vi "sub_NI_Vsion_clamp_copy.vi"(7 "Settings":T3={"Contrast"=40, "Filter width"=4, "Steepness"=2, "Subsampling Ratio"=5, "Show Search Area"=FALSE, "Show Search Lines"=FALSE, "Show Edges Found"=FALSE, "Show Result"=TRUE}, 8 "error in (no error)":errorcluster, 9 "Coordinate System":T5 {"Measurement System"."Axis Reference" items=["Direct", "Indirect"]; "Measurement System"."Angle (deg)" format="%.2f"; "Measurement System"."Origin"."Y" format="%.2f"; "Measurement System"."Origin"."X" format="%.2f"; "Reference System"."Axis Reference" items=["Direct", "Indirect"]; "Reference System"."Angle (deg)" format="%.2f"; "Reference System"."Origin"."Y" format="%.2f"; "Reference System"."Origin"."X" format="%.2f"}, 10 "Rectangle":T6 {"Rotation" format="%.2f"; "Left" scale=0.0..1024.0; "Right" scale=0.0..1024.0}, 11 "Image":T4) -> (0 "error out":errorcluster, 1 "clamp_result":T2 {"ROI Descriptor out"."Contours"."Type" items=["No Selection", "Point", "Line", "Rectangle", "Oval", "Polygon", "Freehand Region", "Annulus", "Unused2", "Unused3", "Broken Line", "Freehand Line", "Rotated Rectangle"]}, 2 "dir-data":cluster{"Distance":sgl, "weight-dir":dbl}, 3 "Image Out":T4, 5 "Edge Coordinates":cluster{"X":sgl, "Y":sgl}[](array[cluster]) {"Y" format="%.2f"; "X" format="%.2f"})   [LabVIEW 2019]
uses:
  <vilib>/vision/Image Controls.llb/IMAQ Image.ctl
  Ctrl/clamp-result_cmd.ctl
  <vilib>/vision/NI_Vision_Development_Module.lvlib
panel:
  out "XY 그래프":cluster{"X":sgl, "Y":sgl}[](graph)
  out "Edge Points":cluster{"X":sgl, "Y":sgl}[](array[cluster])
  out "Elapsed time (ms)":u32
  out "Distance":sgl format="%.2f"
  out "Coordinate System (duplicate)":T5 {"Measurement System"."Axis Reference" items=["Direct", "Indirect"]; "Measurement System"."Angle (deg)" format="%.2f"; "Measurement System"."Origin"."Y" format="%.2f"; "Measurement System"."Origin"."X" format="%.2f"; "Reference System"."Axis Reference" items=["Direct", "Indirect"]; "Reference System"."Angle (deg)" format="%.2f"; "Reference System"."Origin"."Y" format="%.2f"; "Reference System"."Origin"."X" format="%.2f"}
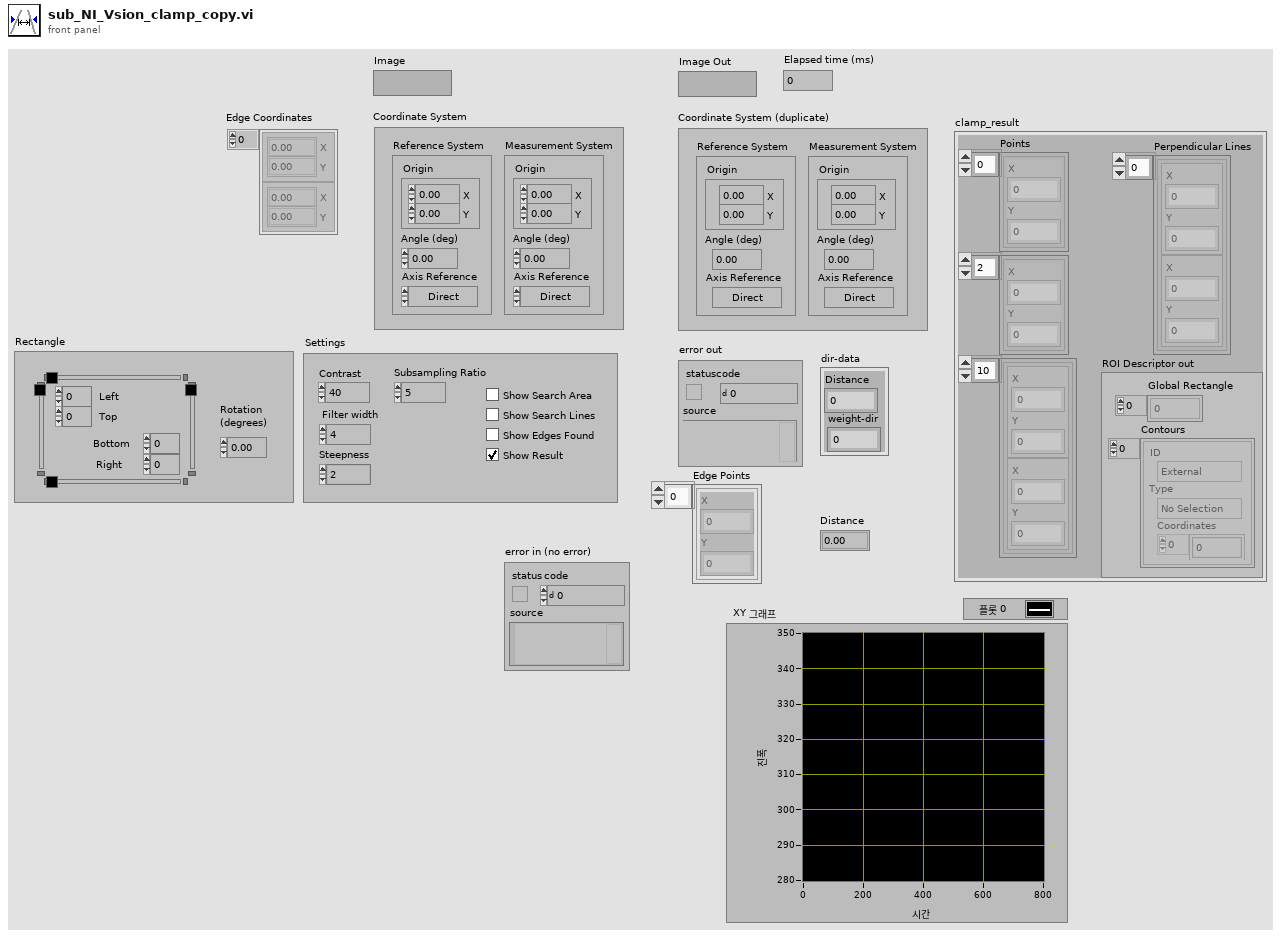
[diagram p1: front panel]
types:
  T1 = typedef "ROI Descriptor" = cluster{"Global Rectangle":i32[], "Contours":cluster{"ID":enum32{"External", "Internal"}, "Type":u32, "Coordinates":i32[]}[]}
  T2 = cluster{"Points":cluster{"X":sgl, "Y":sgl}[], cluster{"X":sgl, "Y":sgl}[], cluster{cluster{"X":sgl, "Y":sgl}, cluster{"X":sgl, "Y":sgl}}[], "Perpendicular Lines":cluster{cluster{"X":sgl, "Y":sgl}, cluster{"X":sgl, "Y":sgl}}[], "ROI Descriptor out":T1}
  T3 = cluster{"Contrast":i32, "Filter width":i32, "Steepness":i32, "Subsampling Ratio":u32, "Show Search Area":bool, "Show Search Lines":bool, "Show Edges Found":bool, "Show Result":bool}
  T4 = typedef "IMAQ Image.ctl" = refnum<image>
  T5 = typedef "IMAQ Coordinate System" = cluster{"Reference System":cluster{"Origin":cluster{"X":sgl, "Y":sgl}, "Angle (deg)":sgl, "Axis Reference":u32}, "Measurement System":cluster{"Origin":cluster{"X":sgl, "Y":sgl}, "Angle (deg)":sgl, "Axis Reference":u32}}
  T6 = typedef "IMAQ Rectangle" = cluster{"Left":i32, "Top":i32, "Right":i32, "Bottom":i32, "Rotation":dbl}
  T7 = typedef "clamp-result_cmd.ctl" = enum16{"write_clamp_overlay-result", "write_center-distance", "write_clamp_result", "write_threshold_result", "read"}
  T8 = cluster{"Origin":cluster{"X":sgl, "Y":sgl}, "Angle (deg)":sgl, "Axis Reference":u32}
  T9 = cluster{"Global Rectangle":i32[], "Contours":cluster{"ID":enum32{"External", "Internal"}, "Type":u32, "Coordinates":i32[]}[]}
  T10 = cluster{"Interpolation Type":enum32{"", "Quadratic", "Cubic Spline"}, "SubPixel Accuracy":enum32{"None", "One Half", "One Third", "One Fourth", "One Fifth", "One Sixth", "One Seventh", "One Eight", "One Ninth", "One Tenth", "One Eleventh", "One Twelveth"}}
  T11 = enum32{"Get First Edge", "Get First + Last Edge", "Get All Edges"}
  T12 = cluster{"Contrast":i32, "Filter width":i32, "Steepness":i32}
  T13 = cluster{cluster{"X":sgl, "Y":sgl}, cluster{"X":sgl, "Y":sgl}}[]
  T14 = cluster{cluster{"X":sgl, "Y":sgl}, cluster{"X":sgl, "Y":sgl}}
  T15 = cluster{"Show Search Area":bool, "Show Search Lines":bool, "Show Edges Found":bool, "Show Result":bool}
  T16 = cluster{"x-center":dbl, "Image Size":cluster{"x":i32, "y":i32}, "Angle deg":sgl, "Threshold Range":cluster{"Lower value":sgl, "Upper value":sgl}}
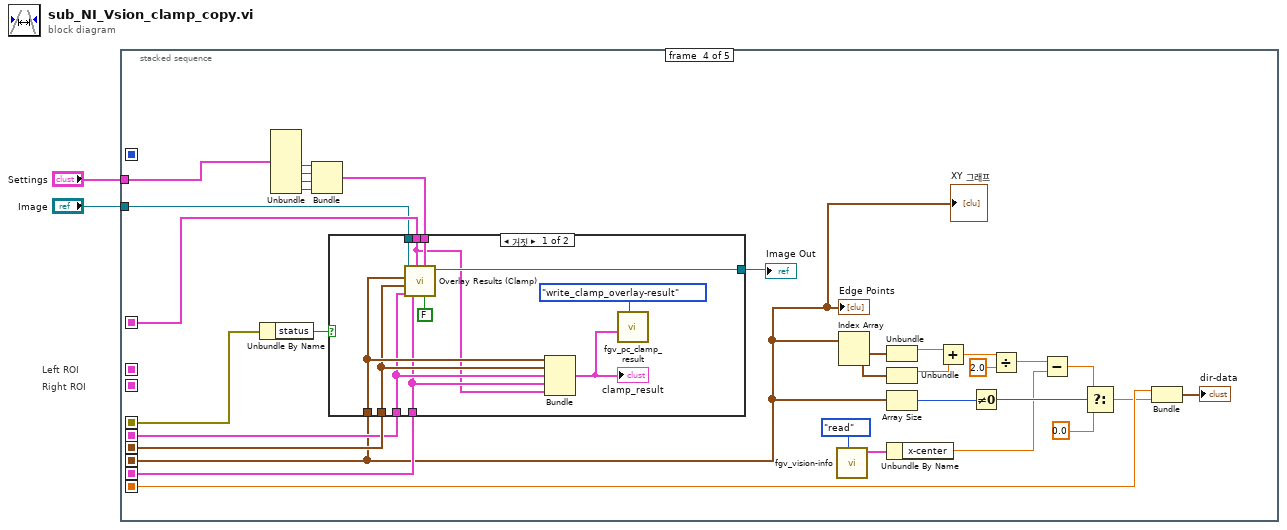
[diagram p0: block diagram]
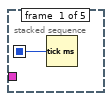
[diagram p2: hidden frame]
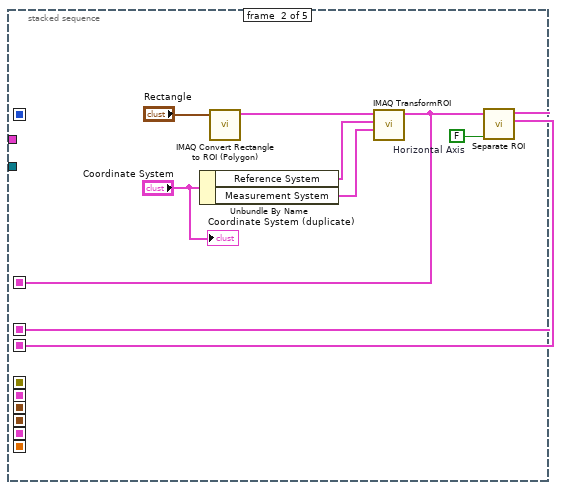
[diagram p3: hidden frame]
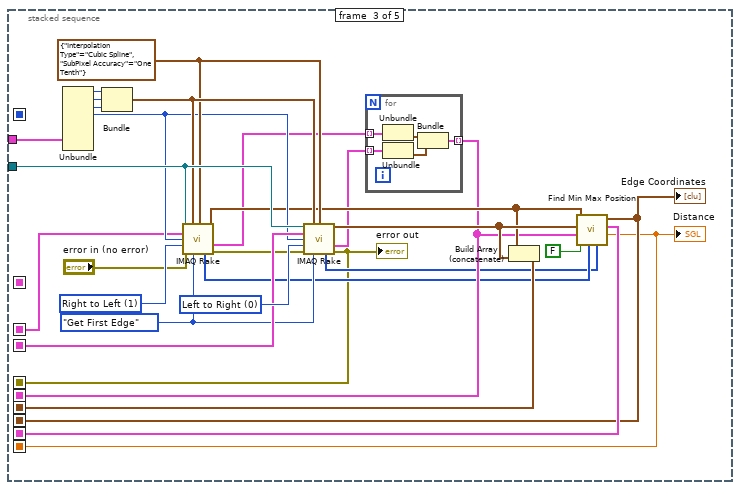
[diagram p4: hidden frame]
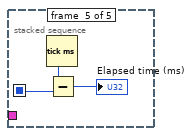
[diagram p6: hidden frame]
diagram:
  # "Right ROI"
  # "Left ROI"
  n1 = stacked-sequence {
    seq-local: [_ _ w33 _ _] -> [_ _ _ w46 _]
    seq-local: [w3 _ _ _ _] -> [_ _ _ _ w92]
    seq-local: [_ _ w34 _ _] -> [_ _ _ w73 _]
    seq-local: [_ _ w20 _ _] -> [_ _ _ w72 _]
    seq-local: [_ _ w37 _ _] -> [_ _ _ w71 _]
    seq-local: [_ w8 _ _ _] -> [_ _ w18 _ _]
    seq-local: [_ w7 _ _ _] -> [_ _ w32 _ _]
    seq-local: [_ w6 _ _ _] -> [_ _ _ w69 _]
    seq-local: [_ _ w14 _ _] -> [_ _ _ w66 _]
    seq-local: [_ _ w13 _ _] -> [_ _ _ w53 _]
    tunnel: "Image" -> [_ _ w30 w68 _]
    tunnel: "Settings" -> [_ _ w17 w50 _]
    frame #0 {
      n2 = Tick Count (ms)() -> (millisecond timer value=w3:u32)
    }
    frame #1 {
      w9 = FALSE  # Horizontal Axis
      # "Find Edges"
      n3 = Unbundle By Name("Coordinate System") -> ("Reference System"=w5:T8, "Measurement System"=w4:T8)
      n4 = call "IMAQ Convert Rectangle to ROI (Polygon)"("Rectangle"="Rectangle") -> ("ROI Descriptor"=w10:T1)  [unwired: 7 in, 2 out]
      n5 = call "IMAQ TransformROI"("New Reference"=w4, "Base Reference"=w5, "ROI Descriptor"=w10) -> ("ROI Descriptor out"=w6:T1)  [unwired: 7 in, 1 out]
      n6 = call <vilib>:"Separate ROI.vi"("Axis"=w9, "ROI Descriptor"=w6) -> ("Right/Bottom ROI"=w7:T9, "Left/Top ROI"=w8:T9)  [unwired: 4 in]
      "Coordinate System (duplicate)" <- "Coordinate System"
    }
    frame #2 {
      w27 = u32 1 items=["Left to Right", "Right to Left", "Top to Bottom", "Bottom to Top"]
      w28 = T10 {"Interpolation Type"=enum."Cubic Spline", "SubPixel Accuracy"=enum."One Tenth"} ("SubPixel Information")
      w22 = T11."Get First Edge" ("Process")
      w35 = u32 0 items=["Left to Right", "Right to Left", "Top to Bottom", "Bottom to Top"]
      # "Find Edges"
      n7 = Unbundle(w17) -> ("Contrast"=w38:i32, "Filter width"=w39:i32, "Steepness"=w40:i32, "Subsampling Ratio"=w25:u32)  [unwired: 4 out]
      n8 = Bundle("Contrast"=w38, "Filter width"=w39, "Steepness"=w40) -> (w29:T12)  [unwired: 1 in]
      n9 = call "IMAQ Rake"("Image"=w30, "Edge Parameters"=w29, "SubPixel Information"=w28, "ROI Descriptor"=w18, "Step Size"=w25, "Scan Direction"=w27, "error in (no error)"="error in (no error)", "Process"=w22) -> ("First Edges"=w23:cluster{"X":sgl, "Y":sgl}[], "Line Coordinates"=w21:T13, "Lines with Edges"=w16:u32[], "error out"=w31:errorcluster)  [unwired: 2 in, 2 out]
      n10 = call "IMAQ Rake"("Image"=w30, "Edge Parameters"=w29, "SubPixel Information"=w28, "ROI Descriptor"=w32, "Step Size"=w25, "Scan Direction"=w35, "error in (no error)"=w31, "Process"=w22) -> ("First Edges"=w24:cluster{"X":sgl, "Y":sgl}[], "Line Coordinates"=w19:T13, "Lines with Edges"=w15:u32[], "error out"=w14:errorcluster)  [unwired: 2 in, 2 out]
      "error out" <- w14
      n11 = for {
        tunnel: w21 -> [w45] mode=indexing
        tunnel: w19 -> [w44] mode=indexing
        tunnel: [w41] -> w20 mode=indexing
        n12 = Unbundle(w45) -> (w43:cluster{"X":sgl, "Y":sgl})  [unwired: 1 out]
        n13 = Unbundle(w44) -> (w42:cluster{"X":sgl, "Y":sgl})  [unwired: 1 out]
        n14 = Bundle(w43, w42) -> (w41:T14)  [unwired: 1 in]
      }
      n15 = Build Array (concatenate)(w23, w24) -> (w34:cluster{"X":sgl, "Y":sgl}[])
      n16 = call <vilib>:"Find Min Max Position.vi"("Lines with Edges (last)"=w15, "Lines with Edges (first)"=w16, "Min / Max"=FALSE, "Search Lines"=w20, "Last Edges"=w24, "First Edges"=w23) -> ("Distance"=w13:sgl, "Perpendicular Lines"=w37:T13, "Points"=w33:cluster{"X":sgl, "Y":sgl}[])  [unwired: 3 in]
      "Edge Coordinates" <- w33
      "Distance" <- w13
    }
    frame #3 {
      # "Update Overlay"
      n17 = Unbundle By Name(w66) -> ("status"=w65:bool)
      n18 = Unbundle(w50) -> ("Show Search Area"=w77:bool, "Show Search Lines"=w76:bool, "Show Edges Found"=w75:bool, "Show Result"=w74:bool)  [unwired: 4 out]
      n19 = Bundle("Show Search Area"=w77, "Show Search Lines"=w76, "Show Edges Found"=w75, "Show Result"=w74) -> (w70:T15)  [unwired: 1 in]
      n20 = case shown="거짓" w65 {
        tunnel: w46 -> [w84 _]
        tunnel: w73 -> [w83 _]
        tunnel: w72 -> [w82 _]
        tunnel: w71 -> [w81 _]
        tunnel: w70 -> [w87 _]
        tunnel: w69 -> [w80 _]
        tunnel: w68 -> [w86 w89]
        tunnel: [w85 w89] -> w67
        frame False {
          n21 = call <vilib>:"Overlay Results (Clamp).vi"("Min / Max"=FALSE, "Setup"=w87, "Perpendicular Lines"=w81, "ROI Descriptor"=w80, "Search Lines"=w82, "All Edges Found"=w83, "Measurement Edges"=w84, "Image In"=w86) -> ("Image Out"=w85:T4)  [unwired: 3 in]
          n22 = Bundle("Points"=w84, w83, w82, "Perpendicular Lines"=w81, "ROI Descriptor out"=w80) -> (w78:T2)  [unwired: 1 in]
          "clamp_result" <- w78
          n23 = call "fgv_pc_clamp_result.vi"("cmd"=clamp-result_cmd."write_clamp_overlay-result", "clamp_roi_overlay-result_in"=w78) -> ()  [unwired: 6 in, 4 out]
        }
        frame True {
        }
      }
      "Image Out" <- w67
      n24 = call "fgv_vision-info.vi"("cmd"=enum16{"read", "write"}."read") -> ("image info out"=w48:T16)  [unwired: 10 in]
      n25 = Index Array(array=w46) -> (element #1=w64:cluster{"X":sgl, "Y":sgl}, element #2=w63:cluster{"X":sgl, "Y":sgl})  [unwired: 2 in]
      n26 = Unbundle(w64) -> ("X"=w62:sgl)  [unwired: 1 out]
      n27 = Unbundle(w63) -> ("X"=w61:sgl)  [unwired: 1 out]
      n28 = Array Size(array=w46) -> (size(s)=w57:i32)
      n29 = Unbundle By Name(w48) -> ("x-center"=w47:dbl)
      n30 = Add(x=w62, y=w61) -> (x+y=w60:sgl)
      n31 = Not Equal To 0?(x=w57) -> (x != 0?=w56:bool)
      n32 = Divide(x=w60, y=sgl 2.0) -> (x/y=w58:sgl)
      n33 = Subtract(x=w58, y=w47) -> (x-y=w54:dbl)
      n34 = Select(t=w54, s=w56, f=0.0 ("t")) -> (s? t:f=w51:dbl)
      n35 = Bundle("Distance"=w53, "t"=w51) -> (→"dir-data":cluster{"Distance":sgl, "t":dbl})  [unwired: 1 in]
      "Edge Points" <- w46
      "XY 그래프" <- w46
    }
    frame #4 {
      n36 = Tick Count (ms)() -> (millisecond timer value=w91:u32)
      n37 = Subtract(x=w91, y=w92) -> (x-y=→"Elapsed time (ms)":u32)
    }
  }
